vi "NF87XX.set position.vi"(0 "i ref in":refnum<vi>, 1 "System":string="N/A", 2 "position":i32, 5 "error in (no error)":errorcluster) -> (14 "i ref out":refnum<vi>, 19 "error out":errorcluster)   [LabVIEW 2014, in "NF87XX.lvlib"]
doc: "Sets the position to move to the active axis.\n\nauthor: Stefan Götte\ndata: 09-JAN-2007\n\n\nLicense Agreement for this software:\n\nCopyright (C)\nGesellschaft für Schwerionenforschung, GSI\nPlanckstr. 1\n64291 Darmstadt\nGermany\n\nContact: D.Beck@gsi.de \n\nThis program is free software; you can redistribute it and/or modify it under the terms of the GNU General Public License as published by the Free Software Foundation; either version 2 of the license, or (at your option) any later version.\n\nThis program is distributed in the hope that it will be useful, but WITHOUT ANY WARRANTY; without even the implied warranty of MERCHANTABILITY or FITNESS FOR A PARTICULAR PURPOSE. See the GNU General License for more details (http://www.gnu.org).\n\nGesellschaft für Schwerionenforschung, GSI\nPlanckstr. 1, 64291 Darmstadt, Germany\nFor all questions and ideas contact: M.Richter@gsi.de, H.Brand@gsi.de or D.Beck@gsi.de.\nLast update: 17-JUN-2004"
uses:
  NF87XX.lvlib
  instr.lib/NewFocusPico/Pico Parameters.ctl
  instr.lib/NewFocusPico/NewFocusPico - Driver np.lvlib
panel:
  in  "Pico Parameter type":T1={"Pico Type"=enum."Open-Loop Pico", "Acceleration (steps/sec^2)"="32000", "Velocity ( Hz)"="2000", "Driver"="A1", "Motor"="0", "Channel"="0", "Process Step"="Final Test"}
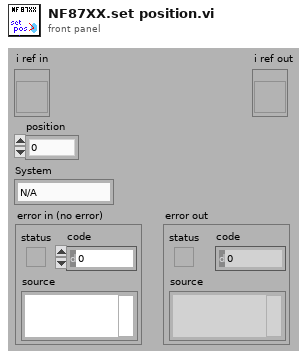
[diagram p1: front panel]
types:
  T1 = typedef "NewFocusPico - Driver np.lvlib/Pico Parameters.ctl" = cluster{"Pico Type":enum16{"Open-Loop Pico", "Close-Loop Pico", "Pico Ultra"}, "Acceleration (steps/sec^2)":string, "Velocity ( Hz)":string, "Driver":string, "Motor":string, "Channel":string, "Process Step":string}
  T2 = typedef "NF87XX.lvlib/NF87XX.driver Type.ctl" = enum16{"not defined", "3-ch open loop drv", "1-ch closed loop drv"}
  T3 = enum16{"User....", "DEF", "DIAG", "INI", "LOCK", "UNLOCK", "MAP", "SAV", "VER", "ACC", "CHL", "FOR", "GO", "HAL", "MOF", "MON", "MPV", "POS", "REL", "REV", "STA", "STO", "TYP", "VEL", "ABS", "SER", "NOS", "DRT", "FLI", "RLI", "FIN", "RIN", "AIN", "IN", "JOF", "JON", "OUT", "RES FINE", "RES COARSE", "02 (HEX)", "PWM", "CNT", "TMR", "HOSTNAME", "IPADDR", "IPMODE", "NETMASK", "GATEWAY", "DNSSRVR", "PASSWD", "ECHO", "MACADDR"}
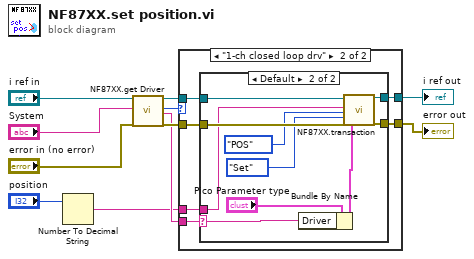
[diagram p0: block diagram]
diagram:
  n1 = Number To Decimal String(number="position") -> (decimal integer string=w2:string)  [unwired: 1 in]
  n2 = call "NF87XX.get Driver.vi"("i ref in"="i ref in", "System"="System", "error in (no error)"="error in (no error)") -> ("i ref out"=w7:refnum<vi>, "Driver Type"=w1:T2, "Driver"=w3:string, "error out"=w6:errorcluster)  [unwired: 12 in, 1 out]
  n3 = case shown="\"1-ch closed loop drv\"" w1 {
    tunnel: [w12 w19] -> w11
    tunnel: [w13 w18] -> w10
    tunnel: w7 -> [w13 w17]
    tunnel: w6 -> [w12 w16]
    tunnel: w3 -> [_ w15]
    tunnel: w2 -> [_ w14]
    frame "not defined", Default {
    }
    frame "1-ch closed loop drv" {
      n4 = case shown="Default" w15 {
        selector: w15 -> [_ w22]
        tunnel: [w20 w31] -> w19
        tunnel: [w21 w30] -> w18
        tunnel: w17 -> [w21 w29]
        tunnel: w16 -> [w20 w28]
        tunnel: w14 -> [_ w27]
        frame "N/A" {
        }
        frame Default {
          n5 = Bundle By Name(cluster="Pico Parameter type", "Driver"=w22) -> (w23:T1)
          n6 = call "NF87XX.transaction.vi"("i ref in"=w29, "User Cmd/Numeric Argu"=w27, "MCL Cmd"=T3."POS", "Query/Set"=enum16{"Query", "Set"}."Set", "error in (no error)"=w28, "Pico Parameter"=w23) -> ("i ref out"=w30:refnum<vi>, "error out"=w31:errorcluster)  [unwired: 11 in, 1 out]
        }
      }
    }
  }
  "error out" <- w11
  "i ref out" <- w10
